vi "ESP32_SHT85_Multi_IP_Acquisition.vi"() -> ()   [LabVIEW 2018]
uses:
  <vilib>/Utility/file.llb/Read Delimited Spreadsheet (string).vi
panel:
  out "Array 2":dbl[][](array[numeric])
  out "Array":string[](array[string])
  in  "UTC":bool
  out "Dernière acquisition":timestamp
  in  "Step (s)":i32=10 min=10 step=1
  out "Liste":cluster{"IP":string, "Statut":bool}[](array[cluster])
  out "Enregistrement en cours":bool
  in  "Start":bool
  in  "Dossier d'enregistrement":path
  out "nb Box":i32
  in  "Stop":bool
  in  "Liste":path
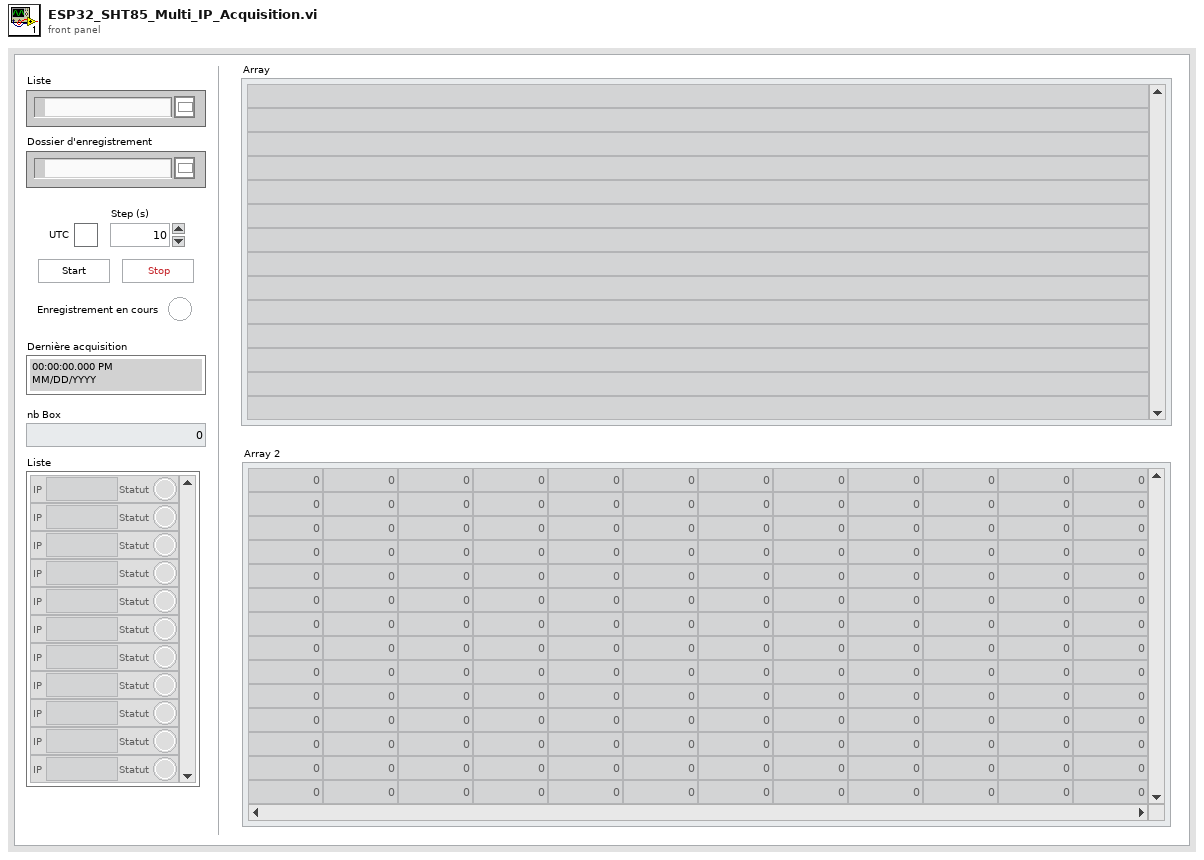
[diagram p1: front panel]
types:
  T1 = enum16{"open", "replace", "create", "open or create", "replace or create", "replace or create with confirmation"}
  T2 = cluster{"Capteur":string, "Temp":dbl, "RH":dbl}[]
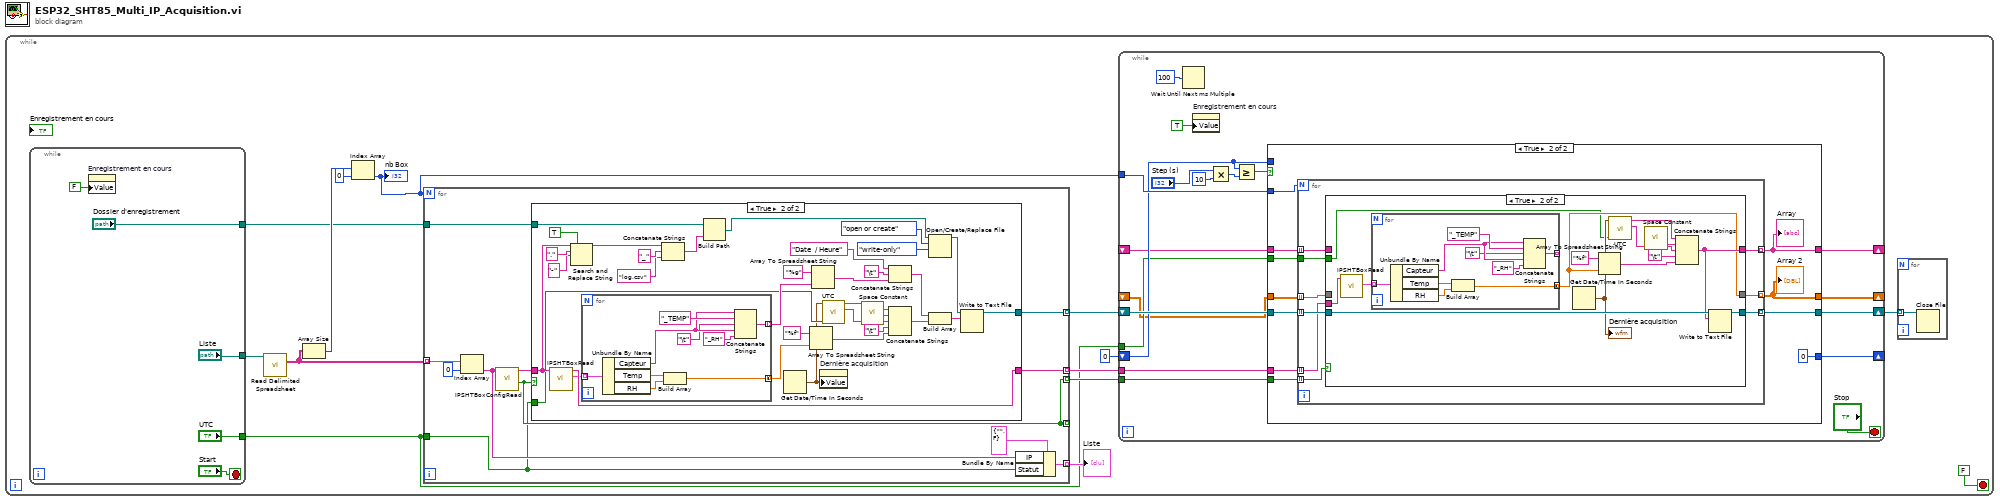
[diagram p0: block diagram]
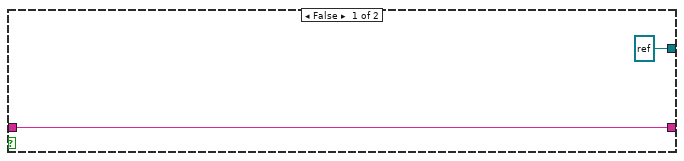
[diagram p2: hidden frame]
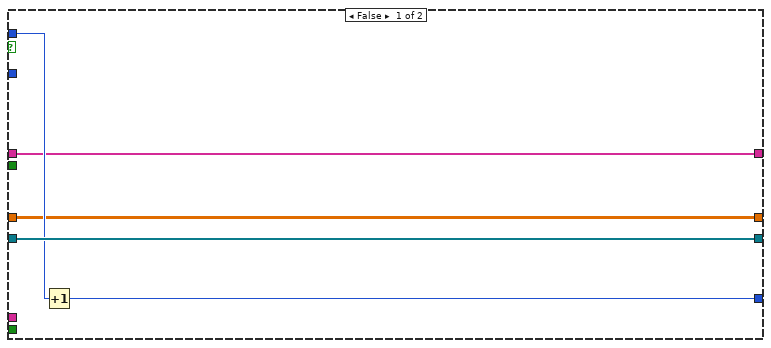
[diagram p3: hidden frame]
diagram:
  n1 = while {
    stop <- FALSE stop-if-true
    n2 = while {
      tunnel: ["Liste"] -> w13
      tunnel: ["Dossier d'enregistrement"] -> w8
      tunnel: ["UTC"] -> w1
      stop <- "Start" stop-if-true
      n3 = property on="Enregistrement en cours" class="Bool (strict)"("Value"=FALSE ("Enregistrement en cours")) -> ()  [unwired: 2 in, 2 out]
    }
    n4 = call-poly <vilib>:"Read Delimited Spreadsheet.vi"("file path (dialog if empty)"=w13) -> ("all rows"=w14:string[][])  [unwired: 9 in, 5 out]
    n5 = Array Size(array=w14) -> (size(s)=w11:i32[])
    n6 = Index Array(array=w11, index=0) -> (element=w9:i32)
    "nb Box" <- w9
    n7 = for {
      N: w9 -> [_]
      tunnel: w14 -> [w31] mode=indexing
      tunnel: [w29] -> w12 mode=indexing
      tunnel: [w25] -> _ mode=indexing
      tunnel: w8 -> [w27]
      tunnel: [w26] -> w7 mode=indexing
      tunnel: w1 -> [w23]
      tunnel: [w25] -> w4 mode=indexing
      tunnel: [w21] -> w2 mode=indexing
      n8 = Index Array(array=w31, index=0) -> (element=w24:string)
      n9 = call "IPSHTBoxConfigRead.vi"("IP in"=w24) -> ("status"=w25:bool, "IP out"=w28:string)  [unwired: 7 in, 2 out]
      n10 = case shown="True" w25 {
        tunnel: [w32 w66] -> w29
        tunnel: w28 -> [w32 w63]
        tunnel: w27 -> [_ w58]
        tunnel: [refnum<file> refnum ("refnum out") w52] -> w26
        tunnel: w23 -> [_ w35]
        frame False {
        }
        frame True {
          n11 = call "IPSHTBoxRead.vi"("IP in"=w63) -> ("cluster"=w51:T2, "IP out"=w66:string)  [unwired: 4 in, 5 out]
          n12 = Search and Replace String(replace all?=TRUE ("replace all? (F)"), input string=w63, search string=".", replace string="-" ("replace string (\"\")")) -> (result string=w59:string)  [unwired: 4 in, 3 out]
          n13 = for {
            tunnel: w51 -> [w75] mode=indexing
            tunnel: [w70] -> w50 mode=indexing
            tunnel: [w67] -> w47 mode=concatenating
            n14 = Unbundle By Name(w75) -> ("Capteur"=w72:string, "Temp"=w69:dbl, "RH"=w68:dbl)
            n15 = Build Array(w69, w68) -> (w67:dbl[])
            n16 = Concatenate Strings(w72, "_TEMP", "\t", w72, "_RH") -> (w70:string)
          }
          n17 = Concatenate Strings(w59, "_", "log.csv") -> (w57:string)
          n18 = Build Path(base path=w58, name or relative path=w57) -> (appended path=w56:path)
          n19 = Get Date/Time In Seconds() -> (seconds since 1Jan1904=w34:timestamp)
          n20 = Array To Spreadsheet String(array=w47, 3:"%f" ("format string")) -> (spreadsheet string=w37:string)  [unwired: 1 in]
          n21 = Array To Spreadsheet String(array=w50, 3:"%g" ("format string")) -> (spreadsheet string=w43:string)  [unwired: 1 in]
          n22 = property on="Dernière acquisition" class="AbsTime (strict)"("Value"=w34) -> ()  [unwired: 2 in, 2 out]
          n23 = call "UTC.vi"("UTC"=w35, "time stamp"=w34) -> ("Heure"=w40:string, "Date"=w41:string)  [unwired: 7 in, 1 out]
          n24 = call <vilib>:"Space Constant.vi"() -> ("String"=w39:string)
          n25 = Concatenate Strings("Date  / Heure" ("string"), "\t", w43) -> (w42:string)
          n26 = Concatenate Strings(w41, w39, w40, "\t", w37) -> (w36:string)
          n27 = Open/Create/Replace File(file path (use dialog)=w56, operation (0:open)=T1."open or create", access (0:read/write)=enum16{"read/write", "read-only", "write-only"}."write-only") -> (refnum out=w53:refnum<file>)  [unwired: 3 in, 2 out]
          n28 = Build Array(w42, w36) -> (w46:string[])
          n29 = Write to Text File(file (use dialog)=w53, text=w46) -> (refnum out=w52:refnum<file>)  [unwired: 2 in, 2 out]
        }
      }
      n30 = Bundle By Name(cluster=cluster{"IP":string, "Statut":bool} {"IP"="", "Statut"=FALSE} ("input cluster"), "IP"=w24, "Statut"=w23) -> (w21:cluster{"IP":string, "Statut":bool})
    }
    "Liste" <- w2
    n31 = while {
      tunnel: w12 -> [w92]
      tunnel: w9 -> [w91]
      tunnel: w4 -> [w87]
      shift-right: [w86] -> _
      shift-left: 0 -> [w83]
      shift-right: [w88] -> w5
      shift-left: w7 -> [w90]
      tunnel: w1 -> [w80]
      shift-right: [w79] -> _
      shift-left: _ -> [w78]
      shift-right: [w77] -> _
      shift-left: _ -> [w76]
      stop <- "Stop" stop-if-true
      n32 = Wait Until Next ms Multiple(millisecond multiple=u32 100) -> ()  [unwired: 1 out]
      n33 = property on="Enregistrement en cours" class="Bool (strict)"("Value"=TRUE ("Enregistrement en cours")) -> ()  [unwired: 2 in, 2 out]
      n34 = Multiply(x="Step (s)", y=10) -> (x*y=w82:i32)
      n35 = Greater Or Equal?(x=w83, y=w82) -> (x >= y?=w81:bool)
      n36 = case shown="True" w81 {
        tunnel: w92 -> [_ w110]
        tunnel: w91 -> [_ w109]
        tunnel: w90 -> [w99 w108]
        tunnel: [w99 w107] -> w88
        tunnel: w87 -> [_ w106]
        tunnel: w83 -> [w98 _]
        tunnel: [w97 0] -> w86
        tunnel: w80 -> [_ w104]
        tunnel: [w96 w103] -> w79
        tunnel: w78 -> [w96 w102]
        tunnel: [w95 w101] -> w77
        tunnel: w76 -> [w95 w100]
        frame False {
          n37 = Increment(x=w98) -> (x+1=w97:i32)
        }
        frame True {
          n38 = for {
            N: w109 -> [_]
            tunnel: w110 -> [w117] mode=indexing
            tunnel: w108 -> [w119] mode=indexing
            tunnel: [w118] -> w107 mode=indexing
            tunnel: w106 -> [w116] mode=indexing
            tunnel: [w115] -> w103 mode=indexing
            tunnel: [w114] -> w101 mode=indexing
            tunnel: w104 -> [w113]
            tunnel: w102 -> [w112] mode=indexing
            tunnel: w100 -> [w111] mode=indexing
            n39 = case shown="True" w116 {
              tunnel: w119 -> [w121 w135]
              tunnel: [w121 w128] -> w118
              tunnel: w117 -> [_ w127]
              tunnel: [w122 w125] -> w115
              tunnel: [w120 w124] -> w114
              tunnel: w113 -> [_ w123]
              tunnel: w112 -> [w122 _]
              tunnel: w111 -> [w120 _]
              frame False {
              }
              frame True {
                n40 = call "IPSHTBoxRead.vi"("IP in"=w127) -> ("cluster"=w126:T2)  [unwired: 4 in, 6 out]
                n41 = for {
                  tunnel: w126 -> [w145] mode=indexing
                  tunnel: [w140] -> _ mode=indexing
                  tunnel: [w137] -> w124 mode=concatenating
                  n42 = Unbundle By Name(w145) -> ("Capteur"=w142:string, "Temp"=w139:dbl, "RH"=w138:dbl)
                  n43 = Build Array(w139, w138) -> (w137:dbl[])
                  n44 = Concatenate Strings(w142, "_TEMP", "\t", w142, "_RH") -> (w140:string)
                }
                n45 = Get Date/Time In Seconds() -> (seconds since 1Jan1904=w134:timestamp)
                "Dernière acquisition" <- w134
                n46 = Array To Spreadsheet String(array=w124, 3:"%f" ("format string")) -> (spreadsheet string=w129:string)  [unwired: 1 in]
                n47 = call "UTC.vi"("UTC"=w123, "time stamp"=w134) -> ("Heure"=w132:string, "Date"=w133:string)  [unwired: 7 in, 1 out]
                n48 = call <vilib>:"Space Constant.vi"() -> ("String"=w131:string)
                n49 = Concatenate Strings(w133, w131, w132, "\t", w129) -> (w125:string)
                n50 = Write to Text File(file (use dialog)=w135, text=w125) -> (refnum out=w128:refnum<file>)  [unwired: 2 in, 2 out]
              }
            }
          }
          "Array" <- w103
          "Array 2" <- w101
        }
      }
    }
    n51 = for {
      tunnel: w5 -> [w15] mode=indexing
      n52 = Close File(refnum=w15) -> ()  [unwired: 1 in, 2 out]
    }
  }
